vi "PS_Laser_Set.vi"(10 "C8 Line?":bool) -> (2 "XY Graph":cluster{dbl[], dbl[]}[](graph), 3 "Voltage Set To":dbl)   [LabVIEW 2011]
uses:
  <vilib>/Utility/error.llb/DialogType.ctl
  <vilib>/DAQmx/write.llb/DAQmx Write (Analog DBL 1Chan 1Samp).vi
  PS_Global.vi
  <vilib>/DAQmx/create/channels.llb/DAQmx Create Channel (AO-Voltage-Basic).vi
  <vilib>/DAQmx/miscellaneous.llb/DAQmx Fill In Error Info.vi
  <vilib>/gmath/NumericalOptimization/Nonlinear Curve Fit LM.vi
  <vilib>/Analysis/NI_AALBase.lvlib
  <vilib>/gmath/NI_Gmath.lvlib
panel:
  out "Voltage 2":dbl
  out "Voltage 1":dbl
  out "best fit parameters":dbl[](array[numeric])
  in  "initial parameters":dbl[](array[numeric])=[0.1, 2.0, 0.5, 0.1, 6.0, 0.5, 5.0]
  out "error out":errorcluster
  in  "termination":cluster{"max iteration":i32, "tolerance":dbl}={"max iteration"=1000, "tolerance"=1e-08}
  in  "Maximum Value 2":dbl=9.9 caption="Maximum Value" format="%0.2f"
  in  "Minimum Value 2":dbl caption="Minimum Value" format="%0.2f"
  out "Voltage for Peak":dbl
  out "max value":dbl
  out "max index(es)":i32
  out "Photodiode Voltage":dbl(graph)
  out "Average Voltage Out":dbl format="%0.2f"
  out "Modulation Voltage":dbl
  out "Votlage Modulation":dbl(graph)
  in  "Minimum Value":dbl=-10.0 format="%0.2f"
  in  "Maximum Value":dbl=10.0 format="%0.2f"
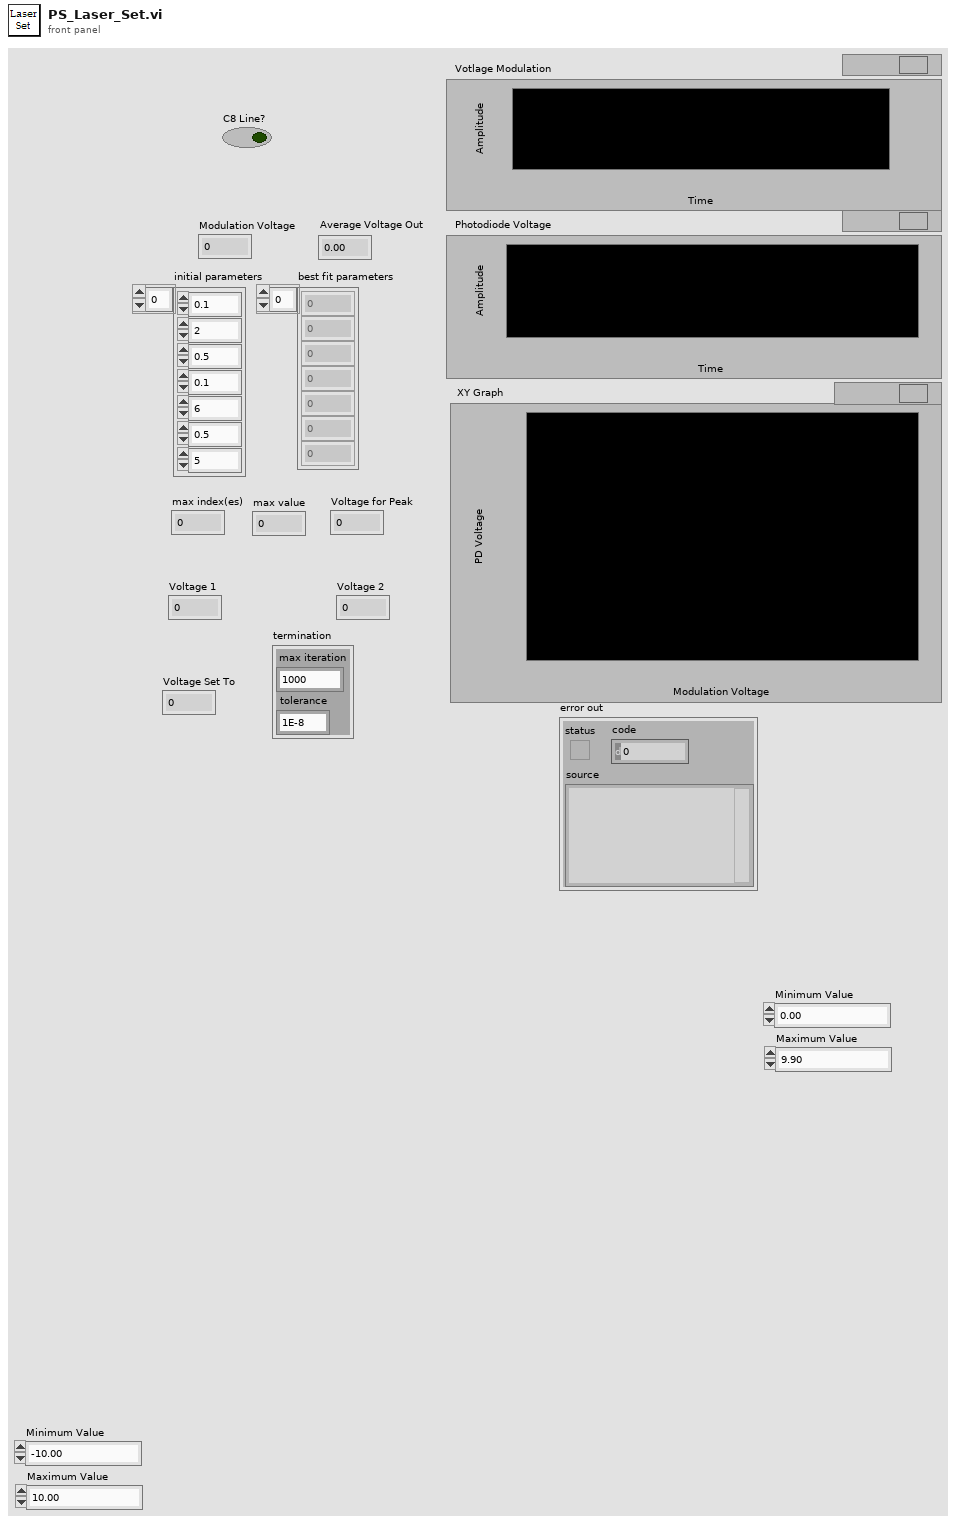
[diagram p1: front panel]
types:
  T1 = typedef "DialogType.ctl" = u16
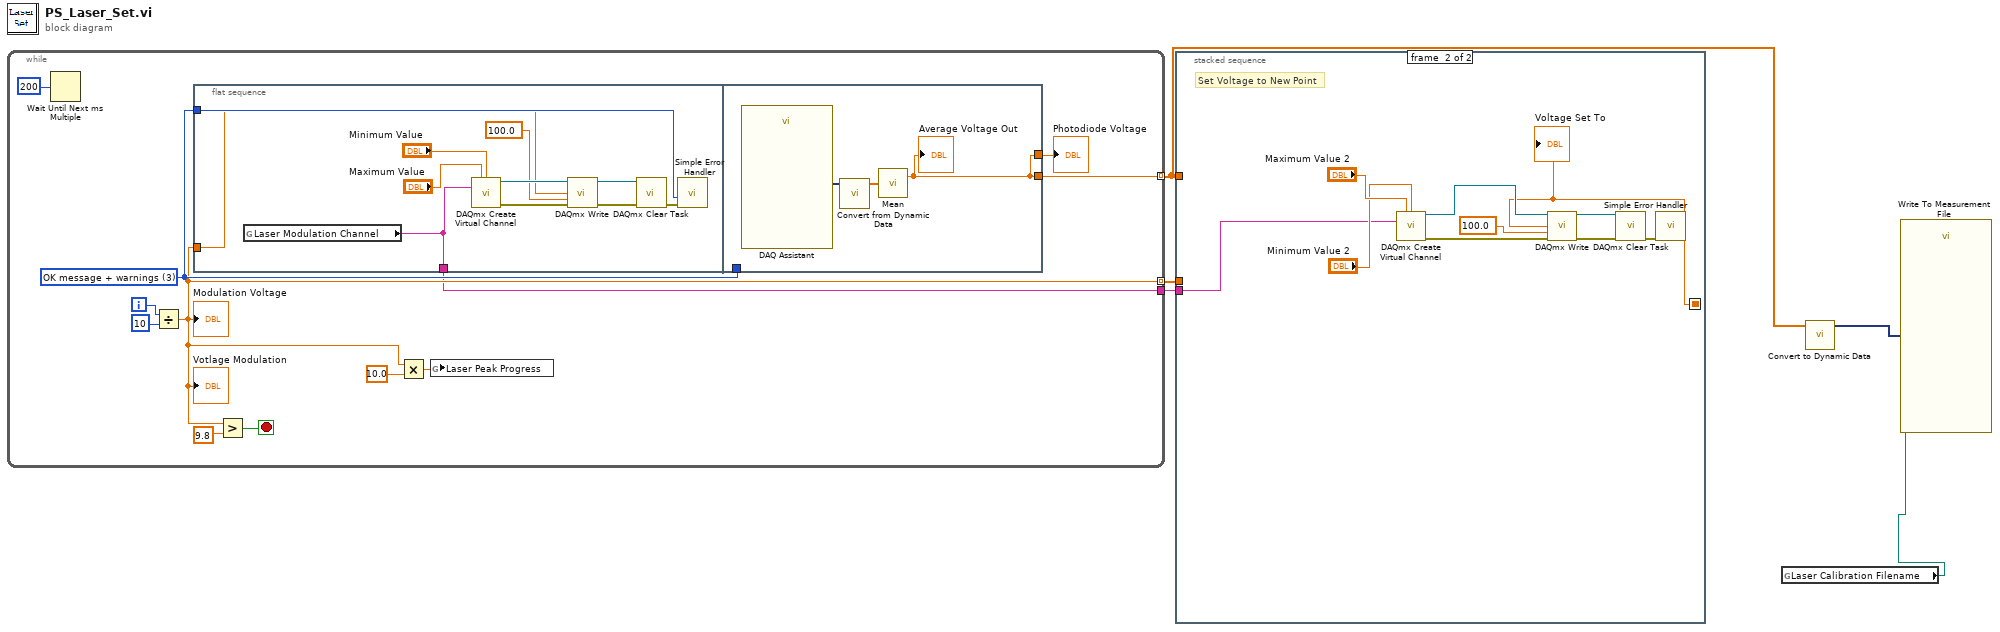
[diagram p0: block diagram]
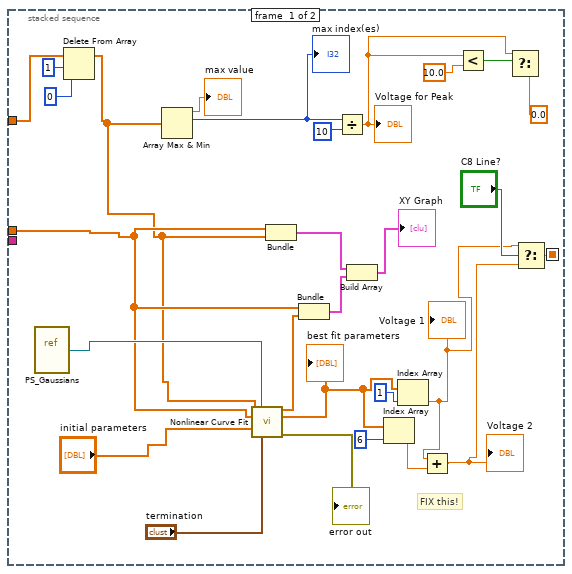
[diagram p2: hidden frame]
diagram:
  n1 = while {
    tunnel: [w10] -> w3 mode=indexing
    tunnel: [w7] -> w5 mode=indexing
    tunnel: [w6] -> w4
    i -> [w16]
    stop <- w13 stop-if-true
    w12 = T1 3 items=["no dialog", "OK message", "continue or stop message", "OK message + warnings", "continue/stop + warnings"] ("type of dialog (OK msg:1)")
    n2 = Wait Until Next ms Multiple(millisecond multiple=u32 200) -> ()  [unwired: 1 out]
    n3 = Divide(x=w16, y=10) -> (x/y=w7:dbl)
    "Votlage Modulation" <- w7
    "Modulation Voltage" <- w7
    n4 = flat-sequence {
      tunnel: w12 -> [w23]
      tunnel: w7 -> [w19]
      tunnel: [w18] -> w6
      tunnel: w12 -> [_]
      tunnel: [w29] -> w11
      tunnel: [w29] -> w10
      frame #0 {
        n5 = global read "PS_Global.vi" "Laser Modulation Channel"() -> (w18:tag)
        n6 = call-poly <vilib>:"DAQmx Create Virtual Channel.vi"("maximum value"="Maximum Value", "minimum value"="Minimum Value", "physical channels"=w18) -> ("task out"=w25:refnum<k21>, "error out"=w26:errorcluster)  [unwired: 11 in]
        n7 = call-poly <vilib>:"DAQmx Write.vi"("task/channels in"=w25, "data"=w19, "timeout"=100.0, "error in"=w26) -> ("task out"=w21:refnum<k21>, "error out"=w22:errorcluster)  [unwired: 9 in, 1 out]
        n8 = call <vilib>:"DAQmx Clear Task.vi"("task in"=w21, "error in"=w22) -> ("error out"=w20:errorcluster)  [unwired: 13 in]
        n9 = call <vilib>:"Simple Error Handler.vi"("type of dialog (OK msg:1)"=w23, "error in (no error)"=w20) -> ()  [unwired: 3 in, 5 out]
      }
      frame #1 {
        n10 = call "DAQ Assistant"() -> ("data"=w30:dynamicdata)  [unwired: 17 in, 2 out]
        n11 = call "Convert from Dynamic Data"("Dynamic Data Type"=w30) -> ("Array"=w31:dbl[])  [unwired: 3 in]
        n12 = call <vilib>:"Mean.vi"("X"=w31) -> ("mean"=w29:dbl)  [unwired: 1 out]
        "Average Voltage Out" <- w29
      }
    }
    n13 = Greater?(x=w7, y=9.8) -> (0:w13:bool)
    n14 = Multiply(x=w7, y=10.0) -> (x*y=w9:dbl)
    n15 = global write "PS_Global.vi" "Laser Peak Progress"(w9) -> ()
    "Photodiode Voltage" <- w11
  }
  n16 = stacked-sequence {
    seq-local: [w42 _] -> [_ w61]
    tunnel: w3 -> [w40 _]
    tunnel: w5 -> [w44 _]
    tunnel: w4 -> [_ w60]
    frame #0 {
      # "FIX this!"
      n17 = vi-ref "PS_Gaussians.vi"() -> (w47:refnum<vi>)
      n18 = Delete From Array(array=w40, length=1, index=0) -> (array with subset deleted=w39:dbl[])  [unwired: 1 out]
      n19 = Array Max & Min(array=w39) -> (max value=→"max value":dbl, max index (indices)=w57:i32)  [unwired: 2 out]
      "max index(es)" <- w57
      n20 = call-poly <vilib>:"Nonlinear Curve Fit.vi"("Y"=w39, "f(x,a)"=w47, "X"=w44, "initial parameters"="initial parameters", "termination"="termination") -> ("best nonlinear fit"=w50:dbl[], "best fit parameters"=w33:dbl[], "error out"=→"error out":errorcluster)  [unwired: 5 in, 3 out]
      "best fit parameters" <- w33
      n21 = Bundle(w44, w39) -> (w52:cluster{dbl[], dbl[]})  [unwired: 1 in]
      n22 = Bundle(w44, "best nonlinear fit"=w50) -> (w45:cluster{dbl[], "best nonlinear fit":dbl[]})  [unwired: 1 in]
      n23 = Divide(x=w57, y=10) -> (x/y=w55:dbl)
      "Voltage for Peak" <- w55
      n24 = Build Array(w52, w45) -> (→"XY Graph":cluster{dbl[], "best nonlinear fit":dbl[]}[])
      n25 = Index Array(array=w33, index=6) -> (element=w34:dbl)
      n26 = Index Array(array=w33, index=1) -> (element=w35:dbl)
      "Voltage 1" <- w35
      n27 = Add(x=w35, y=w34) -> (x+y=w36:dbl)
      "Voltage 2" <- w36
      n28 = Less?(x=w55, y=10.0) -> (x < y?=w53:bool)
      n29 = Select(t=w55, s=w53, f=0.0) -> ()  [unwired: 1 out]
      n30 = Select(t=w35, s="C8 Line?", f=w36) -> (s? t:f=w42:dbl)
    }
    frame #1 {
      # "Set Voltage to New Point"
      n31 = call-poly <vilib>:"DAQmx Create Virtual Channel.vi"("maximum value"="Maximum Value 2", "minimum value"="Minimum Value 2", "physical channels"=w60) -> ("task out"=w65:refnum<k21>, "error out"=w64:errorcluster)  [unwired: 11 in]
      n32 = call-poly <vilib>:"DAQmx Write.vi"("task/channels in"=w65, "data"=w61, "timeout"=100.0, "error in"=w64) -> ("task out"=w68:refnum<k21>, "error out"=w67:errorcluster)  [unwired: 9 in, 1 out]
      n33 = call <vilib>:"DAQmx Clear Task.vi"("task in"=w68, "error in"=w67) -> ("error out"=w69:errorcluster)  [unwired: 13 in]
      n34 = call <vilib>:"Simple Error Handler.vi"("error in (no error)"=w69) -> ()  [unwired: 4 in, 5 out]
      "Voltage Set To" <- w61
    }
  }
  n35 = global read "PS_Global.vi" "Laser Calibration Filename"() -> (w1:path)
  n36 = call "Convert to Dynamic Data"("Array"=w3) -> ("Dynamic Data Type"=w2:dynamicdata)  [unwired: 3 in]
  n37 = call "Write To Measurement File"("Signals"=w2, "Filename"=w1) -> ()  [unwired: 15 in, 3 out]
